vi "SailControlFunction.vi"() -> ()   [LabVIEW 2011]
doc: "Sets the desired sail position based on the apparent wind direction.\nStill under construction."
uses:
  2 Typedefs/apparent wind direction.ctl
  2 Typedefs/sail setpt.ctl
  2 Typedefs/SailLookupTable.ctl
panel:
  in  "Sail Setpoint Lookup Table":T1
  out "Sail Position":T2
  in  "Apparent Wind\nDirection":T3
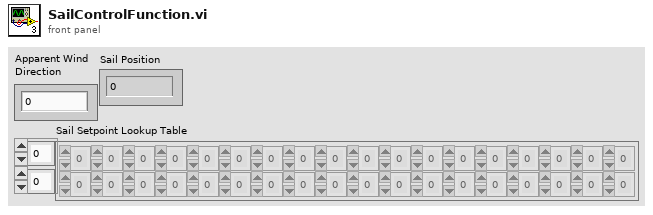
[diagram p1: front panel]
types:
  T1 = typedef "SailLookupTable.ctl" = dbl[][]
  T2 = typedef "sail setpt.ctl" = dbl
  T3 = typedef "apparent wind direction.ctl" = dbl
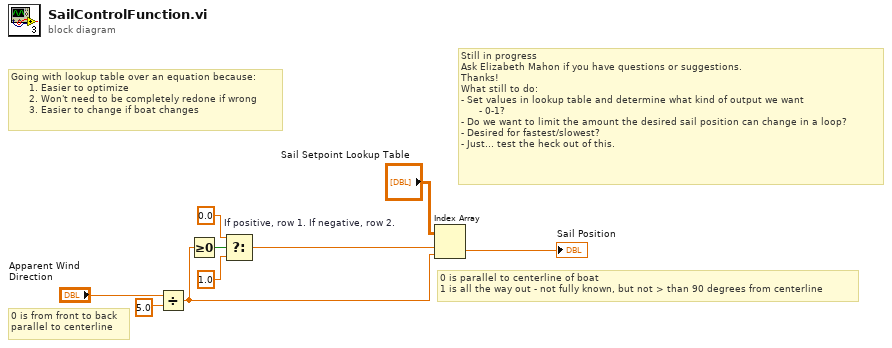
[diagram p0: block diagram]
diagram:
  # "Still in progress\nAsk Elizabeth Mahon if you have questions or suggestions.\nThanks!\nWhat still to do:\n- Set values in lookup table and determine what kind of output we want\n      - 0-1?\n- Do we want to limit the amount the desired sail position can change in a loop?\n- Desired for fastest/slowest?\n- Just... test the heck out of this."
  # "0 is parallel to centerline of boat\n1 is all the way out - not fully known, but not > than 90 degrees from centerline"
  # "0 is from front to back\nparallel to centerline"
  # "Going with lookup table over an equation because:\n      1. Easier to optimize\n      2. Won't need to be completely redone if wrong\n      3. Easier to change if boat changes"
  n1 = Divide(x="Apparent Wind\nDirection", y=T3 5.0) -> (x/y=w2:T3)
  n2 = Greater Or Equal To 0?(x=w2) -> (x >= 0?=w6:bool)
  n3 = Select "If positive, row 1. If negative, row 2."(t=0.0, s=w6, f=1.0) -> (s? t:f=w3:dbl)
  n4 = Index Array(array="Sail Setpoint Lookup Table", index (row)=w3, index (col)=w2) -> (element=→"Sail Position":dbl)
